vi "Delete States.vi"(0 "Tosca in":refnum<class "Parameters.lvclass">, 5 "stateIndex":i32[](array[numeric])) -> (4 "Tosca out":refnum<class "Parameters.lvclass">)   [LabVIEW 2020, in "Parameters.lvclass"]
uses:
  Parameters.lvclass
  Parameters.lvclass/Parameters.ctl
  State/State.lvclass/State.ctl
  State/Read Name.vi
  State/State.lvclass
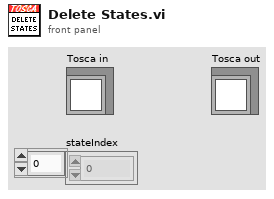
[diagram p1: front panel]
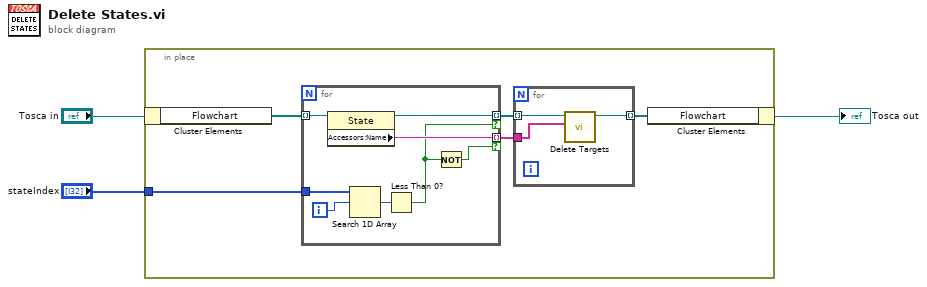
[diagram p0: block diagram]
diagram:
  n1 = in-place {
    in-place-border: "stateIndex" -> [w7]
    n2 = in-place-cluster #1("Tosca in") -> ("Flowchart"=w8:refnum<class "State.lvclass">[])
    n3 = for {
      tunnel: w8 -> [w16] mode=indexing
      tunnel: [w15] -> w4 mode=indexing if=w13
      tunnel: w7 -> [w19]
      tunnel: [w14] -> w6 mode=indexing if=w12
      i -> [w18]
      n4 = property class="State"(reference=w16) -> (reference out=w15:refnum<class "State.lvclass">, "Accessors:Name"=w14:string)  [unwired: 1 in, 1 out]
      n5 = Search 1D Array(1D array=w19, element=w18) -> (index of element=w17:i32)  [unwired: 1 in]
      n6 = Less Than 0?(x=w17) -> (x < 0?=w13:bool)
      n7 = Not(x=w13) -> (.not. x?=w12:bool)
    }
    n8 = for {
      tunnel: w4 -> [w11] mode=indexing
      tunnel: w6 -> [w10]
      tunnel: [w9] -> w5 mode=indexing
      n9 = call "Delete Targets.vi"("Targets"=w10, "State in"=w11) -> ("State out"=w9:refnum<class "State.lvclass">)  [unwired: 8 in, 1 out]
    }
    n10 = in-place-cluster #1("Flowchart"=w5) -> (→"Tosca out":refnum<class "Parameters.lvclass">)
  }
